vi "Error File Logger.vi"(0 "errlog Name":string="Errors.log", 1 "Module":string, 2 "Clear Error?":bool=TRUE, 3 "ContainerFolder(Empty for Application Folder)":path, 5 "error in (no error)":errorcluster) -> (4 "Error Log":string, 6 "error out":errorcluster)   [LabVIEW 2014]
uses:
  <userlib>/_OpenG.lib/file/file.llb/Valid Path - Traditional__ogtk.vi
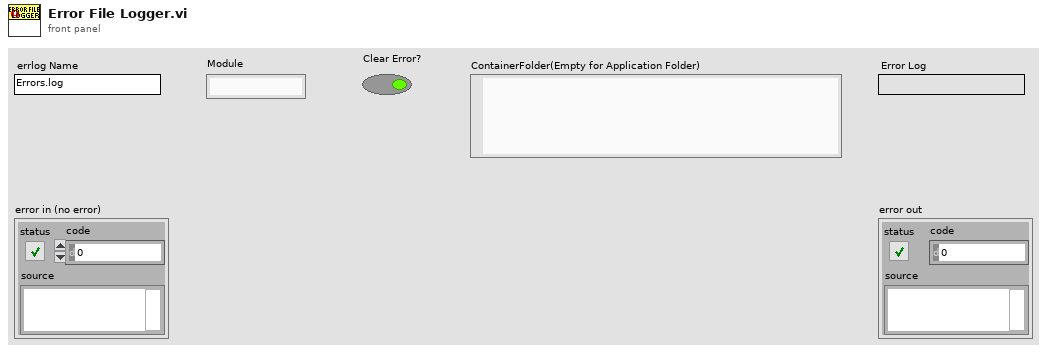
[diagram p1: front panel]
types:
  T1 = enum16{"open", "replace", "create", "open or create", "replace or create", "replace or create with confirmation"}
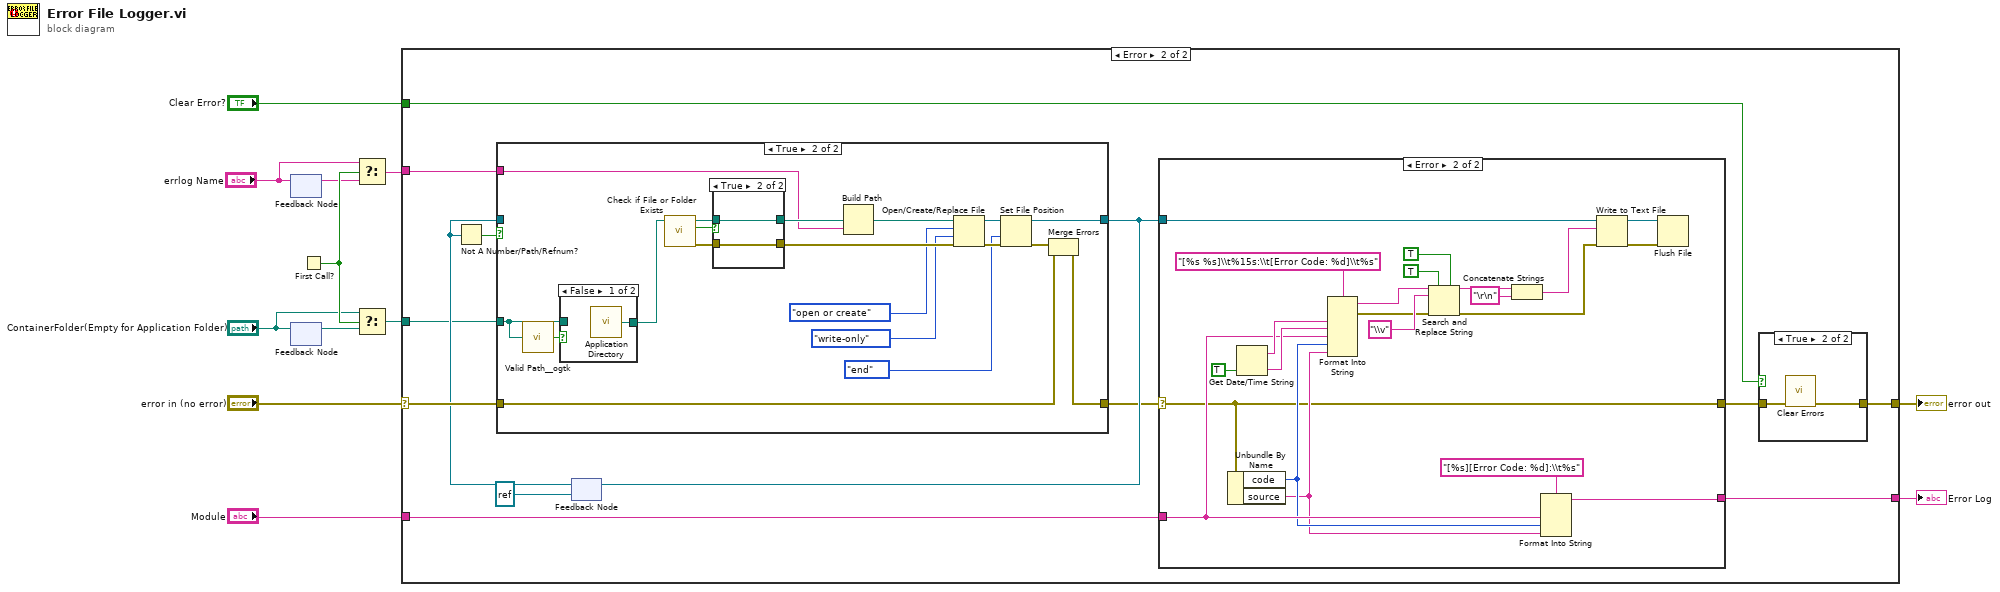
[diagram p0: block diagram]
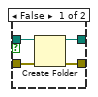
[diagram p7: hidden frame]
diagram:
  n1 = feedback-in #1("errlog Name") -> ()
  n2 = feedback #1() -> (w5:string)  [unwired: 1 in]
  n3 = feedback #2() -> (w6:path)  [unwired: 1 in]
  n4 = feedback-in #2("ContainerFolder(Empty for Application Folder)") -> ()
  n5 = First Call?() -> (First Call?: T/F=w7:bool)
  n6 = Select(t="errlog Name", s=w7, f=w5) -> (s? t:f=w3:string)
  n7 = Select(t="ContainerFolder(Empty for Application Folder)", s=w7, f=w6) -> (s? t:f=w2:path)
  n8 = case shown="Error" "error in (no error)" {
    selector: "error in (no error)" -> [w13 w26]
    tunnel: "Module" -> [_ w20]
    tunnel: [w13 w15] -> w10
    tunnel: w3 -> [_ w22]
    tunnel: [_ w17] -> w9
    tunnel: w2 -> [_ w16]
    tunnel: "Clear Error?" -> [_ w14]
    frame No Error {
    }
    frame Error {
      n9 = feedback #3(refnum<file> refnum ("Error Log File Refnum")) -> (w24:refnum<file>)
      n10 = Not A Number/Path/Refnum?(number/path/refnum=w24) -> (NaN/Path/Refnum?=w25:bool)
      n11 = case shown="True" w25 {
        tunnel: w26 -> [w53 w57]
        tunnel: [w53 w58] -> w19
        tunnel: [w54 w61] -> w21
        tunnel: w24 -> [w54 _]
        tunnel: w22 -> [_ w59]
        tunnel: w16 -> [_ w55]
        frame False {
        }
        frame True {
          n12 = call-poly <userlib>:"Valid Path__ogtk.vi"("path"=w55) -> ("valid"=w56:bool)
          n13 = case shown="False" w56 {
            tunnel: [w74 w75] -> w68
            tunnel: w55 -> [_ w75]
            frame False {
              n14 = call <vilib>:"Application Directory.vi"() -> ("Application Directory"=w74:path)
            }
            frame True {
            }
          }
          n15 = call <vilib>:"Check if File or Folder Exists.vi"("path"=w68) -> ("error out"=w73:errorcluster, "file or folder exists?"=w69:bool, "dup path"=w71:path)  [unwired: 8 in]
          n16 = case shown="True" w69 {
            tunnel: w73 -> [w79 w80]
            tunnel: [w78 w80] -> w70
            tunnel: w71 -> [w77 w81]
            tunnel: [w76 w81] -> w72
            frame False {
              n17 = Create Folder(path (use dialog)=w77, error in=w79) -> (created path=w76:path, error out=w78:errorcluster)  [unwired: 1 in, 1 out]
            }
            frame True {
            }
          }
          n18 = Build Path(base path=w72, name or relative path=w59) -> (appended path=w65:path)
          n19 = Open/Create/Replace File(file path (use dialog)=w65, error in=w70, operation (0:open)=T1."open or create", access (0:read/write)=enum16{"read/write", "read-only", "write-only"}."write-only") -> (refnum out=w64:refnum<file>, error out=w63:errorcluster)  [unwired: 2 in, 1 out]
          n20 = Set File Position(refnum=w64, from (0:start)=enum16{"start", "end", "current"}."end", error in=w63) -> (refnum out=w61:refnum<file>, error out=w60:errorcluster)  [unwired: 1 in]
          n21 = Merge Errors(w60, w57) -> (w58:errorcluster)
        }
      }
      n22 = feedback-in #3(w21) -> ()
      n23 = case shown="Error" w19 {
        selector: w19 -> [w30 w31]
        tunnel: w21 -> [_ w38]
        tunnel: w20 -> [_ w35]
        tunnel: [_ w32] -> w17
        tunnel: [w30 w31] -> w18
        frame No Error {
        }
        frame Error {
          n24 = Unbundle By Name(w31) -> ("code"=w34:i32, "source"=w33:string)
          n25 = Get Date/Time String(want seconds? (F)=TRUE) -> (date string=w50:string, time string=w49:string)  [unwired: 2 in]
          n26 = Format Into String(format string="[%s %s]\\t%15s:\\t[Error Code: %d]\\t%s", w50, w49, w35, w34, w33) -> (resulting string=w45:string, error out=w43:errorcluster)  [unwired: 2 in]
          n27 = Search and Replace String(replace all?=TRUE ("replace all? (F)"), multiline?=TRUE ("ignore case? (F)"), input string=w45, search string="\\v" ("string"), error in=w43) -> (result string=w37:string, error out=w39:errorcluster)  [unwired: 3 in, 2 out]
          n28 = Concatenate Strings(w37, "\r\n" ("string")) -> (w47:string)
          n29 = Format Into String(format string="[%s][Error Code: %d]:\\t%s", w35, w34, w33) -> (resulting string=w32:string)  [unwired: 2 in, 1 out]
          n30 = Write to Text File(file (use dialog)=w38, text=w47, error in=w39) -> (refnum out=w40:refnum<file>, error out=w48:errorcluster)  [unwired: 1 in, 1 out]
          n31 = Flush File(refnum=w40, error in=w48) -> ()  [unwired: 2 out]
        }
      }
      n32 = case shown="True" w14 {
        tunnel: w18 -> [w27 w29]
        tunnel: [w27 w28] -> w15
        frame False {
        }
        frame True {
          n33 = call <vilib>:"Clear Errors.vi"("error in (no error)"=w29) -> ("error out"=w28:errorcluster)  [unwired: 5 in, 1 out]
        }
      }
    }
  }
  "error out" <- w10
  "Error Log" <- w9
